vi "Auto Fire.vi"(11 "Robot Commands":T1) -> ()   [LabVIEW 2015]
uses:
  Joystick/Robot Commands.ctl
  <vilib>/Rock Robotics/WPI/Solenoid/WPI_SolenoidValue.ctl
  <vilib>/Rock Robotics/WPI/Relay/WPI_RelayValue.ctl
panel:
  out "E-Stop":bool
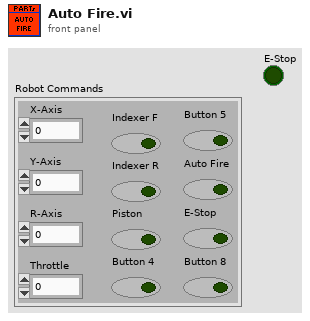
[diagram p1: front panel]
types:
  T1 = typedef "Robot Commands.ctl" = cluster{"X-Axis":dbl, "Y-Axis":dbl, "R-Axis":dbl, "Throttle":dbl, "Indexer F":bool, "Indexer R":bool, "Piston":bool, "Button 4":bool, "Button 5":bool, "Auto Fire":bool, "E-Stop":bool, "Button 8":bool}
  T2 = typedef "WPI_SolenoidValue.ctl" = enum16{"Off", "On", "Forward", "Reverse"}
  T3 = typedef "WPI_RelayValue.ctl" = enum16{"Off", "On", "Forward", "Reverse"}
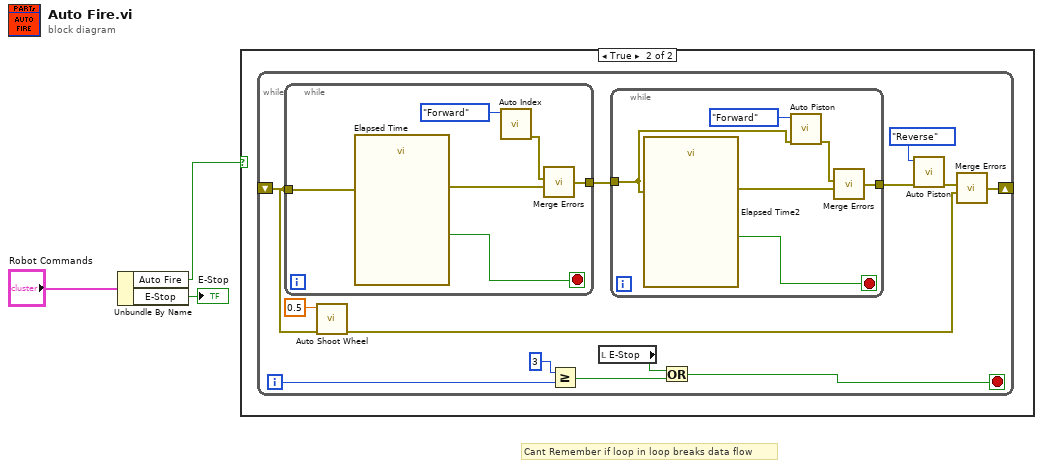
[diagram p0: block diagram]
diagram:
  # "Cant Remember if loop in loop breaks data flow"
  n1 = Unbundle By Name("Robot Commands") -> ("Auto Fire"=w3:bool, "E-Stop"=→"E-Stop":bool)
  n2 = case shown="True" w3 {
    frame False {
    }
    frame True {
      n3 = while {
        shift-right: [w12] -> _
        shift-left: _ -> [w4]
        i -> [w10]
        stop <- w7 stop-if-true
        n4 = while {
          tunnel: [w24] -> w5
          tunnel: w4 -> [w23]
          stop <- w28 stop-if-true
          n5 = call "Elapsed Time"("error in (no error)"=w23) -> ("Time has Elapsed"=w28:bool, "error out"=w25:errorcluster)  [unwired: 11 in, 6 out]
          n6 = call "Auto Index.vi"("RelayValue"=WPI_RelayValue."Forward") -> ("error out"=w26:errorcluster)  [unwired: 10 in]
          n7 = call "Merge Errors.vi"("error in 2"=w25, "error in"=w26) -> ("error out"=w24:errorcluster)  [unwired: 2 in]
        }
        n8 = call "Auto Shoot Wheel.vi"("error in (no error)"=w4, "Output"=0.5) -> ("error out"=w14:errorcluster)  [unwired: 9 in]
        n9 = Greater Or Equal?(x=3, y=w10) -> (x >= y?=w8:bool)
        n10 = local read "E-Stop"() -> (w6:bool)
        n11 = while {
          tunnel: w5 -> [w20]
          tunnel: [w17] -> w15
          stop <- w22 stop-if-true
          n12 = call "Elapsed Time2"("error in (no error)"=w20) -> ("Time has Elapsed"=w22:bool, "error out"=w18:errorcluster)  [unwired: 11 in, 6 out]
          n13 = call "Auto Piston.vi"("error in (no error)"=w20, "Value"=WPI_SolenoidValue."Forward") -> ("error out"=w19:errorcluster)  [unwired: 9 in]
          n14 = call "Merge Errors.vi"("error in 2"=w18, "error in"=w19) -> ("error out"=w17:errorcluster)  [unwired: 2 in]
        }
        n15 = Or(x=w6, y=w8) -> (x .or. y?=w7:bool)
        n16 = call "Auto Piston.vi"("error in (no error)"=w15, "Value"=WPI_SolenoidValue."Reverse") -> ("error out"=w13:errorcluster)  [unwired: 9 in]
        n17 = call "Merge Errors.vi"("error in 2"=w14, "error in"=w13) -> ("error out"=w12:errorcluster)  [unwired: 2 in]
      }
    }
  }
